vi "readScreenBmp subvi.vi"(7 "Numeric":i32, 8 "error in (no error)":errorcluster, 9 "file name":string, 10 "base path":path, 11 "TCP Network Connection in":refnum<k5>) -> (3 "new picture":picture)   [LabVIEW 2013]
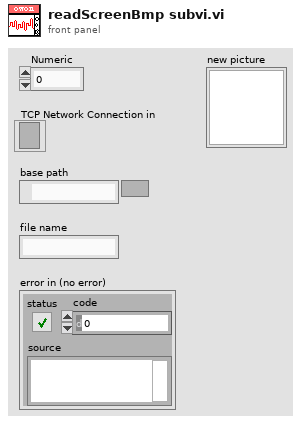
[diagram p1: front panel]
types:
  T1 = enum16{"Standard", "Buffered", "CRLF", "Immediate"}
  T2 = typedef "imagedata.ctl" = cluster{"image type":i32, "image depth":i32, "image":u8[], "mask":u8[], "colors":u32[], "Rectangle":cluster{"left":i16, "top":i16, "right":i16, "bottom":i16}}
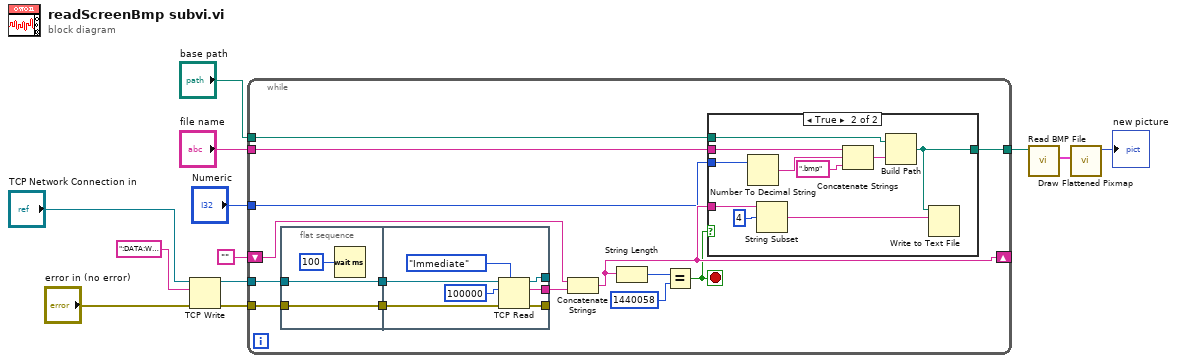
[diagram p0: block diagram]
diagram:
  n1 = TCP Write(connection ID="TCP Network Connection in", data in=":DATA:WAVE:SCREEN:BMP?" ("ID Query"), error in (no error)="error in (no error)") -> (connection ID out=w2:refnum<k5>, error out=w3:errorcluster)  [unwired: 1 in, 1 out]
  n2 = while {
    tunnel: w2 -> [w24]
    tunnel: w3 -> [w23]
    shift-right: [w18] -> _
    shift-left: "" -> [w22]
    tunnel: "Numeric" -> [w16]
    tunnel: [w15] -> w6
    tunnel: "file name" -> [w14]
    tunnel: "base path" -> [w13]
    stop <- w17 stop-if-true
    n3 = flat-sequence {
      tunnel: [w39] -> w26
      tunnel: [w38] -> w25
      tunnel: w24 -> [w39]
      tunnel: w23 -> [w38]
      tunnel: [w46] -> _
      tunnel: [w45] -> _
      tunnel: w26 -> [w44]
      tunnel: w25 -> [w43]
      tunnel: [w40] -> w21
      frame #0 {
        n4 = Wait (ms)(milliseconds to wait=u32 100) -> ()  [unwired: 1 out]
      }
      frame #1 {
        n5 = TCP Read(connection ID=w44, bytes to read=u32 100000 ("byte count"), error in (no error)=w43, 7:T1."Immediate" ("mode (standard)")) -> (connection ID out=w46:refnum<k5>, data out=w40:string, error out=w45:errorcluster)  [unwired: 1 in]
      }
    }
    n6 = Concatenate Strings(w22, w21) -> (w18:string)
    n7 = String Length(string=w18) -> (length=w20:i32)
    n8 = Equal?(x=w20, y=1440058) -> (x = y?=w17:bool)
    n9 = case shown="True" w17 {
      tunnel: w18 -> [_ w32]
      tunnel: w16 -> [_ w30]
      tunnel: [_ w29] -> w15
      tunnel: w14 -> [_ w28]
      tunnel: w13 -> [_ w27]
      frame False {
      }
      frame True {
        n10 = Number To Decimal String(number=w30) -> (decimal integer string=w33:string)  [unwired: 1 in]
        n11 = String Subset(string=w32, offset (0)=4 ("偏移量(0)")) -> (substring=w36:string)  [unwired: 1 in]
        n12 = Concatenate Strings(w28, w33, ".bmp" ("Substring")) -> (w34:string)
        n13 = Build Path(base path=w27, name or relative path=w34) -> (appended path=w29:path)
        n14 = Write to Text File(file (use dialog)=w29, text=w36) -> ()  [unwired: 2 in, 3 out]
      }
    }
  }
  n15 = call <vilib>:"Read BMP File.vi"("path to BMP file"=w6) -> ("image data"=w7:T2)  [unwired: 8 in, 2 out]
  n16 = call <vilib>:"Draw Flattened Pixmap.vi"("image data"=w7) -> ("new picture"=→"new picture":picture)  [unwired: 8 in]
